vi "copyright.vi"(2 "year":u16) -> ()   [LabVIEW 2015]
uses:
  toolbar icons/help.ctl
  <vilib>/Platform/browser.llb/Open URL in Default Browser (string).vi
panel:
  in  "Help Button":T1
  in  "OK Button":bool
  out "Info":string
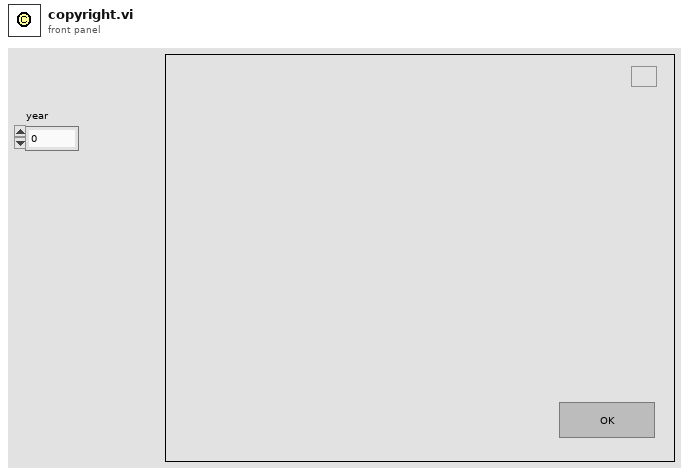
[diagram p1: front panel]
types:
  T1 = typedef "help.ctl" = bool
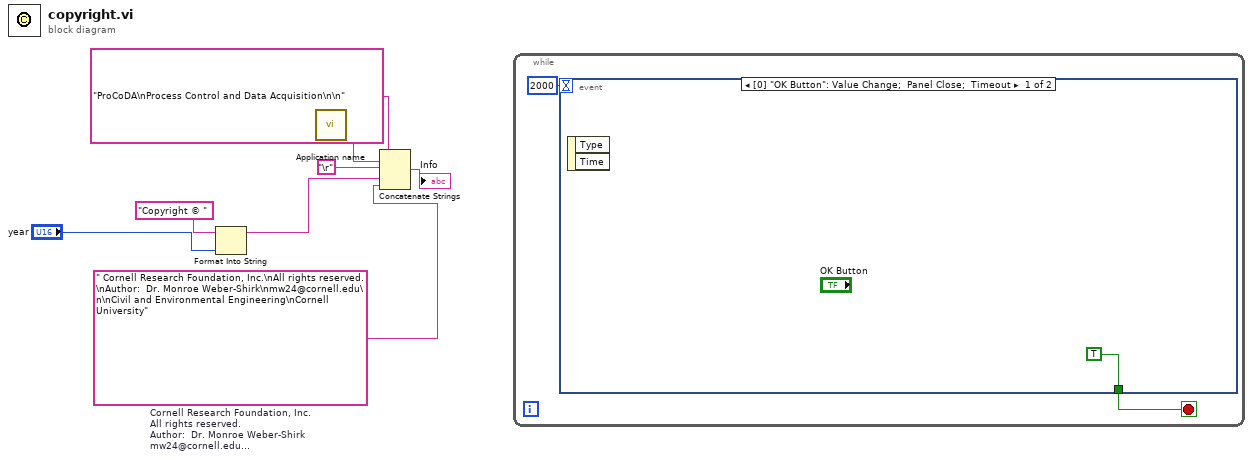
[diagram p0: block diagram]
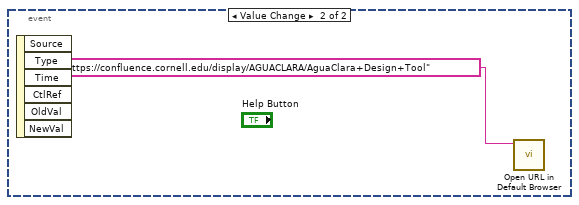
[diagram p2: hidden frame]
diagram:
  w5 = " Cornell Research Foundation, Inc.\nAll rights reserved.\nAuthor:  Dr. Monroe Weber-Shirk\nmw24@cornell.edu\n\nCivil and Environmental Engineering\nCornell University"  # Cornell Research Foundation, Inc. All rights reserved. Author:  Dr. Monroe Weber-Shirk mw24@cornell.edu  Civil and Environmental Engineering Cornell University
  n1 = Format Into String(initial string="Copyright © ", "year") -> (resulting string=w6:string)  [unwired: 2 in, 1 out]
  n2 = call "Application name.vi"() -> ("application name"=w3:string)  [unwired: 5 in, 2 out]
  n3 = Concatenate Strings("ProCoDA\nProcess Control and Data Acquisition\n\n" ("string"), w3, "\r", w6, w5) -> (→"Info":string)
  n4 = while {
    stop <- w10 stop-if-true
    n5 = event shown="[0] \"OK Button\": Value Change;  Panel Close;  Timeout" {
      selector: _ -> [_ _]
      dyn-events: _ -> [_ _]
      timeout: 2000 -> [_ _]
      tunnel: [TRUE _] -> w10
      event "OK Button": Value Change; Panel Close; Timeout {
        n6 = event-data() -> ()  [unwired: 1 in, 2 out]
      }
      event Value Change {
        n7 = event-data() -> ()  [unwired: 1 in, 6 out]
        n8 = call-poly <vilib>:"Open URL in Default Browser.vi"("URL"="https://confluence.cornell.edu/display/AGUACLARA/AguaClara+Design+Tool") -> ()  [unwired: 5 in, 2 out]
      }
    }
  }
